vi "geve-update_config_file.vi"(8 "error in (no error)":errorcluster, 10 "Serial Port Configuration":T1={"timeout (ms)"=0, "VISA resource name"="", "baud rate"=0, "max expected byte count"=128}) -> (0 "error out":errorcluster, 1 "serial cfg":T1={"timeout (ms)"=0, "VISA resource name"="", "baud rate"=0, "max expected byte count"=128}, 2 "info":string)   [LabVIEW 2018]
doc: "Get serial configuration and write it to the config.ini file"
uses:
  geve-serial_config_cluster.ctl
  <vilib>/Utility/config.llb/Write Key (String).vi
  <vilib>/Utility/config.llb/Write Key (U32).vi
  <vilib>/Utility/config.llb/Read Key (String).vi
  <vilib>/Utility/config.llb/Read Key (I32).vi
  <vilib>/Utility/config.llb/NI_LVConfig.lvlib
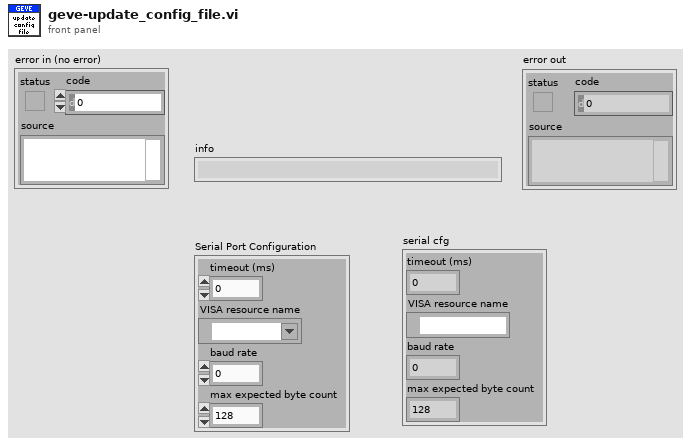
[diagram p1: front panel]
types:
  T1 = typedef "geve-serial_config_cluster.ctl" = cluster{"timeout (ms)":u32, "VISA resource name":refnum<visa-resource-name>, "baud rate":u32, "max expected byte count":u32}
  T2 = typedef "NI_LVConfig.lvlib/Config Data RefNum.ctl" = refnum<k1>
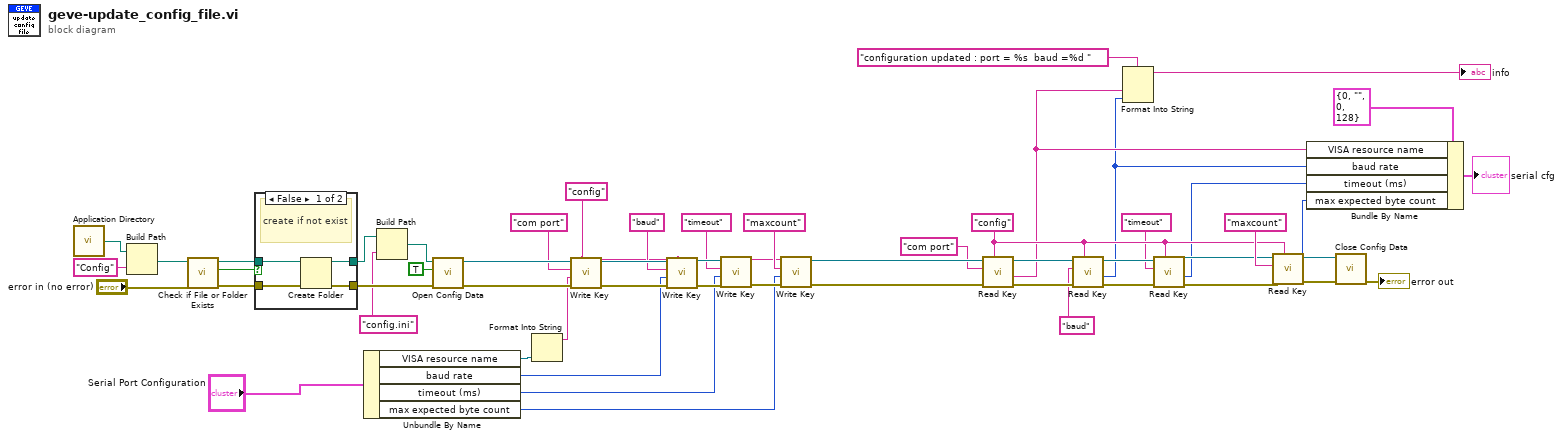
[diagram p0: block diagram]
diagram:
  w10 = "config" ("section")
  w26 = "config" ("section")
  n1 = call <vilib>:"Application Directory.vi"() -> ("Application Directory"=w54:path)
  n2 = Build Path(base path=w54, name or relative path="Config") -> (appended path=w52:path)
  n3 = call <vilib>:"Check if File or Folder Exists.vi"("error in (no error)"="error in (no error)", "path"=w52) -> ("error out"=w47:errorcluster, "file or folder exists?"=w51:bool, "dup path"=w50:path)  [unwired: 7 in]
  n4 = case shown="False" w51 {
    tunnel: w50 -> [w59 w61]
    tunnel: [w58 w61] -> w38
    tunnel: [w56 w60] -> w48
    tunnel: w47 -> [w57 w60]
    frame False {
      # "create if not exist"
      n5 = Create Folder(path (use dialog)=w59, error in=w57) -> (created path=w58:path, error out=w56:errorcluster)  [unwired: 1 in, 1 out]
    }
    frame True {
    }
  }
  n6 = Unbundle By Name("Serial Port Configuration") -> ("VISA resource name"=w3:refnum<visa-resource-name>, "baud rate"=w4:u32, "timeout (ms)"=w6:u32, "max expected byte count"=w5:u32)
  n7 = Build Path(base path=w38, name or relative path="config.ini") -> (appended path=w35:path)
  n8 = call <vilib>:"Open Config Data.vi"("error in (no error)"=w48, "create file if necessary (T)"=TRUE, "configuration file path"=w35) -> ("error out"=w45:errorcluster, "refnum"=w49:T2)  [unwired: 6 in, 1 out]
  n9 = Format Into String(w3) -> (resulting string=w2:string)  [unwired: 3 in, 1 out]
  n10 = call-poly <vilib>:"Write Key.vi"("section"=w10, "error in (no error)"=w45, "value"=w2, "key"="com port", "refnum"=w49) -> ("error out"=w15:errorcluster, "refnum out"=w18:T2)  [unwired: 4 in, 1 out]
  n11 = call-poly <vilib>:"Write Key.vi"("section"=w10, "error in (no error)"=w15, "value"=w4, "key"="baud", "refnum"=w18) -> ("error out"=w13:errorcluster, "refnum out"=w14:T2)  [unwired: 4 in, 1 out]
  n12 = call-poly <vilib>:"Write Key.vi"("section"=w10, "error in (no error)"=w13, "value"=w6, "key"="timeout", "refnum"=w14) -> ("error out"=w9:errorcluster, "refnum out"=w8:T2)  [unwired: 4 in, 1 out]
  n13 = call-poly <vilib>:"Write Key.vi"("section"=w10, "error in (no error)"=w9, "value"=w5, "key"="maxcount", "refnum"=w8) -> ("error out"=w42:errorcluster, "refnum out"=w43:T2)  [unwired: 4 in, 1 out]
  n14 = call-poly <vilib>:"Read Key.vi"("section"=w26, "error in (no error)"=w42, "key"="com port", "refnum"=w43) -> ("error out"=w41:errorcluster, "value"=w23:string, "refnum out"=w44:T2)  [unwired: 4 in, 1 out]
  n15 = call-poly <vilib>:"Read Key.vi"("section"=w26, "error in (no error)"=w41, "key"="baud", "refnum"=w44) -> ("error out"=w30:errorcluster, "value"=w22:i32, "refnum out"=w31:T2)  [unwired: 4 in, 1 out]
  n16 = Format Into String(format string="configuration updated : port = %s  baud =%d " ("section"), w23, w22) -> (resulting string=→"info":string)  [unwired: 2 in, 1 out]
  n17 = call-poly <vilib>:"Read Key.vi"("section"=w26, "error in (no error)"=w30, "key"="timeout", "refnum"=w31) -> ("error out"=w29:errorcluster, "value"=w21:i32, "refnum out"=w32:T2)  [unwired: 4 in, 1 out]
  n18 = call-poly <vilib>:"Read Key.vi"("section"=w26, "error in (no error)"=w29, "key"="maxcount", "refnum"=w32) -> ("error out"=w28:errorcluster, "value"=w20:i32, "refnum out"=w27:T2)  [unwired: 4 in, 1 out]
  n19 = Bundle By Name(cluster=T1 {"timeout (ms)"=0, "VISA resource name"="", "baud rate"=0, "max expected byte count"=128} ("Serial Port Configuration"), "VISA resource name"=w23, "baud rate"=w22, "timeout (ms)"=w21, "max expected byte count"=w20) -> (→"serial cfg":T1)
  n20 = call <vilib>:"Close Config Data.vi"("error in (no error)"=w28, "refnum"=w27) -> ("error out"=→"error out":errorcluster)  [unwired: 8 in, 1 out]
